vi "macro_Rotation2d_AngleDeg.vi"   [LabVIEW 2019, in "Trajectory_Library.lvlib"]
uses:
  Conv_Deg_Radians.vi
  Rotation2d_CreateAngle.vi
  Rotation2d_GetAngleCosSin.vi
  Trajectory_Library.lvlib
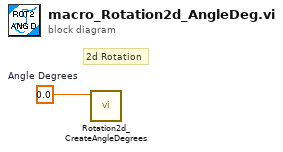
[diagram p0: block diagram]
diagram:
  w1 = 0.0  # Angle Degrees
  # "2d Rotation"
  n1 = call "Rotation2d_CreateAngleDegrees.vi"("Angle_Degrees"=w1) -> ()  [unwired: 10 in, 1 out]
